vi "SPD.Get Results.vi"(4 "ParameterSelector":i32, 5 "SurfaceSelector":i32, 6 "View Selector":i32, 7 "GraphSelector":i32, 8 "Error In":errorcluster, 10 "SPD.Parameter Selector":T2, 11 "SPD.Stand Ctrl in":T3 {"spdDeviceSession"."hidSPD.Controller"."HV_bias" format="%#_6p, V"; "spdDeviceSession"."hidSPD.Controller"."TSet" format="%#_6p, DegC"}) -> (0 "Error Out":errorcluster, 1 "SPD.Surface Plot":T1, 2 "Graph Result":cluster{"HV_Bias":dbl[], dbl[]}[](array[cluster]), 3 "SPD.Stand Ctrl out":T3 {"spdDeviceSession"."hidSPD.Controller"."HV_bias" format="%#_6p, V"; "spdDeviceSession"."hidSPD.Controller"."TSet" format="%#_6p, DegC"})   [LabVIEW 2018]
uses:
  typedefs/SPD.Stand Ctrl.ctl
  Instruments/SPD HID Interface/hidSPDLibForLabView/LibVIs/hidSPD Controls/hidSPD Device Session.ctl
  Instruments/SPD HID Interface/hidSPDLibForLabView/LibVIs/hidSPD Controls/hidSPD Controller.ctl
  Instruments/KC705 DevBoard/typedefs/DevB.Session.ctl
  Instruments/KeySight 53230A/typedefs/FreqC.Session.ctl
  Instruments/KeySight 8164B/KeySight 8164B LAN InstrLib/typedefs/KeySight 8164B control.ctl
  Instruments/LeCroy SDA830/typedefs/LeCroy.Session.ctl
  typedefs/SPD.Events.ctl
  <vilib>/Utility/config.llb/Config Data RefNum.ctl
  typedefs/SPD.Meas Result.ctl
  SPD.Params Selectors.ctl
  SPD.Surface Plot.ctl
  Instruments/SPD HID Interface/hidSPDLibForLabView/hidSPDLibForLabView.lvlib
  Instruments/KeySight 8164B/KeySight 8164B LAN InstrLib.lvlib
  <vilib>/Utility/config.llb/NI_LVConfig.lvlib
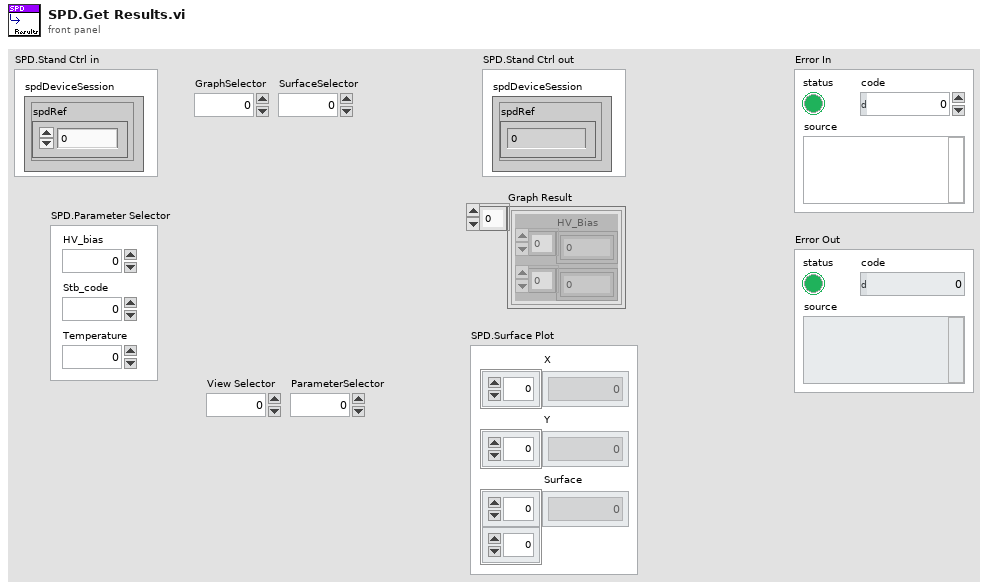
[diagram p1: front panel]
types:
  T1 = typedef "SPD.Surface Plot.ctl" = cluster{"X":dbl[], "Y":dbl[], "Surface":dbl[][]}
  T2 = typedef "SPD.Params Selectors.ctl" = cluster{"HV_bias":i32, "Stb_code":i32, "Temperature":i32}
  T3 = typedef "SPD.Stand Ctrl.ctl" = cluster{"spdDeviceSession":T4, "DevBSession":T6, "FreqCSession":T7, "8164BSession":T8, "LeCroySession":T9, "Events":T10, "configFile":T11, "SPD.Result":T12}
  T4 = typedef "hidSPDLibForLabView.lvlib/hidSPD Device Session.ctl" = cluster{"spdRef":u64, "connected":bool, "spdName":string, "hidSPD.Controller":T5}
  T5 = typedef "hidSPDLibForLabView.lvlib/hidSPD Controller.ctl" = cluster{"TSet":sgl, "HV_bias":sgl, "DDS_stb_code":u16}
  T6 = typedef "DevB.Session.ctl" = cluster{"DevBRef":refnum<visa-resource-name>, "connected":bool}
  T7 = typedef "FreqC.Session.ctl" = cluster{"FreqCRef":refnum<visa-resource-name>, "timeout":dbl, "connected":bool}
  T8 = typedef "KeySight 8164B LAN InstrLib.lvlib/KeySight 8164B control.ctl" = cluster{"Connection ID":refnum<k5>, "Connected":bool, "Info":string, "Slots Info":string[]}
  T9 = typedef "LeCroy.Session.ctl" = cluster{"LeCroySession":refnum<visa-resource-name>, "connected":bool}
  T10 = typedef "SPD.Events.ctl" = cluster{"DCRTest":refnum<user-event>, "Stop":refnum<user-event>}
  T11 = typedef "NI_LVConfig.lvlib/Config Data RefNum.ctl" = refnum<k1>
  T12 = typedef "SPD.Meas Result.ctl" = cluster{"HV_Bias":dbl[], "Stb_code":dbl[], "Temprature":dbl[], "Data":dbl[][][][]}
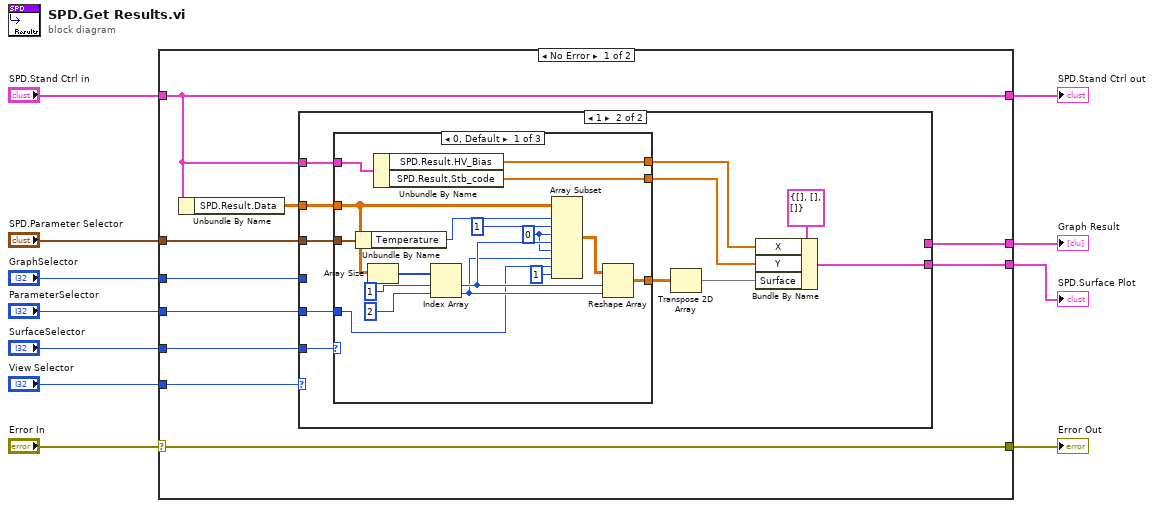
[diagram p0: block diagram]
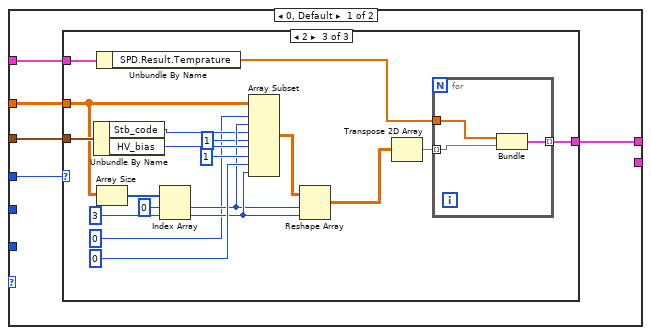
[diagram p2: hidden frame]
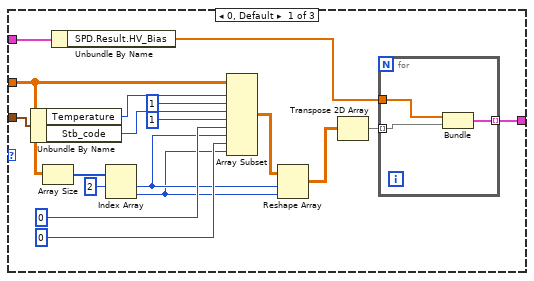
[diagram p3: hidden frame]
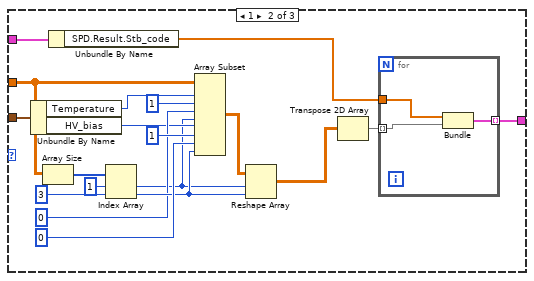
[diagram p4: hidden frame]
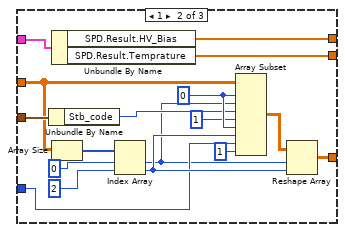
[diagram p5: hidden frame]
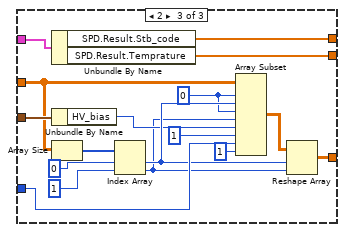
[diagram p6: hidden frame]
diagram:
  n1 = case shown="No Error" "Error In" {
    selector: "Error In" -> [w16 w155]
    tunnel: [w16 w155] -> w10
    tunnel: "SPD.Stand Ctrl in" -> [w15 w154]
    tunnel: [w15 w154] -> w8
    tunnel: "SPD.Parameter Selector" -> [w19 _]
    tunnel: "GraphSelector" -> [w20 _]
    tunnel: [w18 _] -> w4
    tunnel: "View Selector" -> [w17 _]
    tunnel: "SurfaceSelector" -> [w14 _]
    tunnel: "ParameterSelector" -> [w13 _]
    tunnel: [w12 _] -> w1
    frame No Error {
      n2 = Unbundle By Name(w15) -> ("SPD.Result.Data"=w21:dbl[][][][])
      n3 = case shown="1" w17 {
        tunnel: w21 -> [w26 w102]
        tunnel: w20 -> [w25 _]
        tunnel: w19 -> [w24 w100]
        tunnel: [w23 _] -> w18
        tunnel: w15 -> [w22 w101]
        tunnel: w14 -> [_ w99]
        tunnel: w13 -> [_ w98]
        tunnel: [_ w93] -> w12
        frame 0, Default {
          n4 = case shown="2" w25 {
            tunnel: w26 -> [w37 w62 w86]
            tunnel: w24 -> [w44 w66 w88]
            tunnel: [w27 w53 w77] -> w23
            tunnel: w22 -> [w30 w56 w80]
            frame 0, Default {
              n5 = Unbundle By Name(w44) -> ("Temperature"=w43:i32, "Stb_code"=w42:i32)
              n6 = Array Size(array=w37) -> (size(s)=w36:i32[])
              n7 = Unbundle By Name(w30) -> ("SPD.Result.HV_Bias"=w28:dbl[])
              n8 = Index Array(array=w36, index #1=2 ("index")) -> (element #1=w33:i32, element #2=w32:i32)  [unwired: 1 in]
              n9 = Array Subset(array=w37, index (dim 0)=w43, length (dim 0)=1 ("length"), index (dim 1)=w42, length (dim 1)=1 ("length"), index (dim 2)=0 ("index"), length (dim 2)=w33, index (dim 3)=0 ("index"), length (dim 3)=w32) -> (w34:dbl[][][][])
              n10 = Reshape Array(w34, w33, w32) -> (w31:dbl[][])
              n11 = Transpose 2D Array(2D array=w31) -> (transposed array=w29:dbl[][])
              n12 = for {
                tunnel: w29 -> [w46] mode=indexing
                tunnel: w28 -> [w47]
                tunnel: [w45] -> w27 mode=indexing
                n13 = Bundle("HV_Bias"=w47, w46) -> (w45:cluster{"HV_Bias":dbl[], dbl[]})  [unwired: 1 in]
              }
            }
            frame 1 {
              n14 = Unbundle By Name(w66) -> ("Temperature"=w65:i32, "HV_bias"=w49:i32)
              n15 = Array Size(array=w62) -> (size(s)=w61:i32[])
              n16 = Unbundle By Name(w56) -> ("SPD.Result.Stb_code"=w54:dbl[])
              n17 = Index Array(array=w61, index #1=1 ("index"), index #2=3 ("index")) -> (element #1=w48:i32, element #2=w58:i32)
              n18 = Array Subset(array=w62, index (dim 0)=w65, length (dim 0)=1 ("length"), index (dim 1)=0 ("index"), length (dim 1)=w48, index (dim 2)=w49, length (dim 2)=1 ("length"), index (dim 3)=0 ("index"), length (dim 3)=w58) -> (w59:dbl[][][][])
              n19 = Reshape Array(w59, w48, w58) -> (w57:dbl[][])
              n20 = Transpose 2D Array(2D array=w57) -> (transposed array=w55:dbl[][])
              n21 = for {
                tunnel: w55 -> [w68] mode=indexing
                tunnel: w54 -> [w69]
                tunnel: [w67] -> w53 mode=indexing
                n22 = Bundle("Stb_code"=w69, w68) -> (w67:cluster{"Stb_code":dbl[], dbl[]})  [unwired: 1 in]
              }
            }
            frame 2 {
              n23 = Unbundle By Name(w88) -> ("Stb_code"=w71:i32, "HV_bias"=w74:i32)
              n24 = Unbundle By Name(w80) -> ("SPD.Result.Temprature"=w78:dbl[])
              n25 = Array Size(array=w86) -> (size(s)=w85:i32[])
              n26 = Index Array(array=w85, index #1=0 ("index"), index #2=3 ("index")) -> (element #1=w73:i32, element #2=w82:i32)
              n27 = Array Subset(array=w86, index (dim 0)=0 ("index"), length (dim 0)=w73, index (dim 1)=w71, length (dim 1)=1 ("length"), index (dim 2)=w74, length (dim 2)=1 ("length"), index (dim 3)=0 ("index"), length (dim 3)=w82) -> (w83:dbl[][][][])
              n28 = Reshape Array(w83, w73, w82) -> (w81:dbl[][])
              n29 = Transpose 2D Array(2D array=w81) -> (transposed array=w79:dbl[][])
              n30 = for {
                tunnel: w79 -> [w90] mode=indexing
                tunnel: w78 -> [w91]
                tunnel: [w89] -> w77 mode=indexing
                n31 = Bundle("Temprature"=w91, w90) -> (w89:cluster{"Temprature":dbl[], dbl[]})  [unwired: 1 in]
              }
            }
          }
        }
        frame 1 {
          n32 = case shown="0, Default" w99 {
            tunnel: w102 -> [w116 w135 w152]
            tunnel: w100 -> [w119 w136 w153]
            tunnel: w101 -> [w113 w132 w149]
            tunnel: w98 -> [w107 w128 w146]
            tunnel: [w105 w126 w144] -> w96
            tunnel: [w104 w125 w143] -> w95
            tunnel: [w103 w124 w142] -> w94
            frame 0, Default {
              w108 = 0 ("index")
              n33 = Unbundle By Name(w119) -> ("Temperature"=w118:i32)
              n34 = Array Size(array=w116) -> (size(s)=w115:i32[])
              n35 = Unbundle By Name(w113) -> ("SPD.Result.HV_Bias"=w105:dbl[], "SPD.Result.Stb_code"=w104:dbl[])
              n36 = Index Array(array=w115, index #1=1 ("index"), index #2=2 ("index")) -> (element #1=w110:i32, element #2=w109:i32)
              n37 = Array Subset(array=w116, index (dim 0)=w118, length (dim 0)=1 ("length"), index (dim 1)=w108, length (dim 1)=w110, index (dim 2)=w108, length (dim 2)=w109, index (dim 3)=w107, length (dim 3)=1 ("length")) -> (w114:dbl[][][][])
              n38 = Reshape Array(w114, w110, w109) -> (w103:dbl[][])
            }
            frame 1 {
              w123 = 0 ("index")
              n39 = Unbundle By Name(w136) -> ("Stb_code"=w122:i32)
              n40 = Unbundle By Name(w132) -> ("SPD.Result.HV_Bias"=w126:dbl[], "SPD.Result.Temprature"=w125:dbl[])
              n41 = Array Size(array=w135) -> (size(s)=w134:i32[])
              n42 = Index Array(array=w134, index #1=0 ("index"), index #2=2 ("index")) -> (element #1=w120:i32, element #2=w129:i32)
              n43 = Array Subset(array=w135, index (dim 0)=w123, length (dim 0)=w120, index (dim 1)=w122, length (dim 1)=1 ("length"), index (dim 2)=w123, length (dim 2)=w129, index (dim 3)=w128, length (dim 3)=1 ("length")) -> (w133:dbl[][][][])
              n44 = Reshape Array(w133, w120, w129) -> (w124:dbl[][])
            }
            frame 2 {
              w139 = 0 ("index")
              n45 = Unbundle By Name(w149) -> ("SPD.Result.Stb_code"=w144:dbl[], "SPD.Result.Temprature"=w143:dbl[])
              n46 = Unbundle By Name(w153) -> ("HV_bias"=w140:i32)
              n47 = Array Size(array=w152) -> (size(s)=w151:i32[])
              n48 = Index Array(array=w151, index #1=0 ("index"), index #2=1 ("index")) -> (element #1=w141:i32, element #2=w138:i32)
              n49 = Array Subset(array=w152, index (dim 0)=w139, length (dim 0)=w141, index (dim 1)=w139, length (dim 1)=w138, index (dim 2)=w140, length (dim 2)=1 ("length"), index (dim 3)=w146, length (dim 3)=1 ("length")) -> (w150:dbl[][][][])
              n50 = Reshape Array(w150, w141, w138) -> (w142:dbl[][])
            }
          }
          n51 = Transpose 2D Array(2D array=w94) -> (transposed array=w92:dbl[][])
          n52 = Bundle By Name(cluster=T1 {"X"=[], "Y"=[], "Surface"=[]} ("SPD.Surface Plot"), "X"=w96, "Y"=w95, "Surface"=w92) -> (w93:T1)
        }
      }
    }
    frame Error {
    }
  }
  "SPD.Stand Ctrl out" <- w8
  "Error Out" <- w10
  "Graph Result" <- w4
  "SPD.Surface Plot" <- w1
